vi "Test_MO.vi"() -> ()   [LabVIEW 2025]
panel:
  out "Valor 2":bool
  out "Valor":bool
  in  "Pin in":u8=4 min=4 max=40
  in  "Pin 3":u8=4 min=4 max=40
  in  "Pin 2":u8=4 min=4 max=40
  in  "Pin":u8=4 min=4 max=40
  in  "Estado 2":bool
  in  "stop":bool
  in  "VISA resource name":refnum<visa-resource-name>
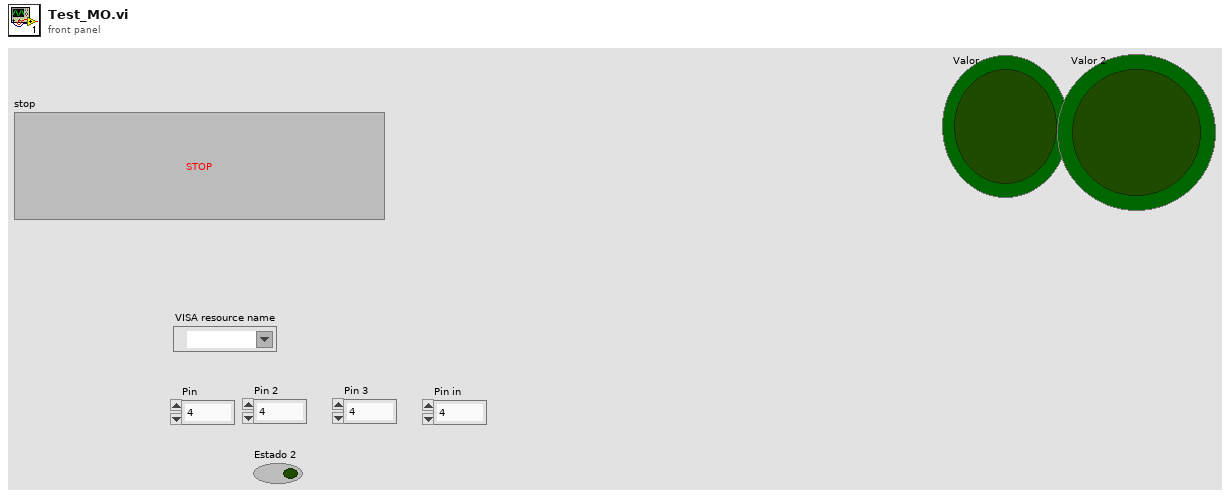
[diagram p1: front panel]
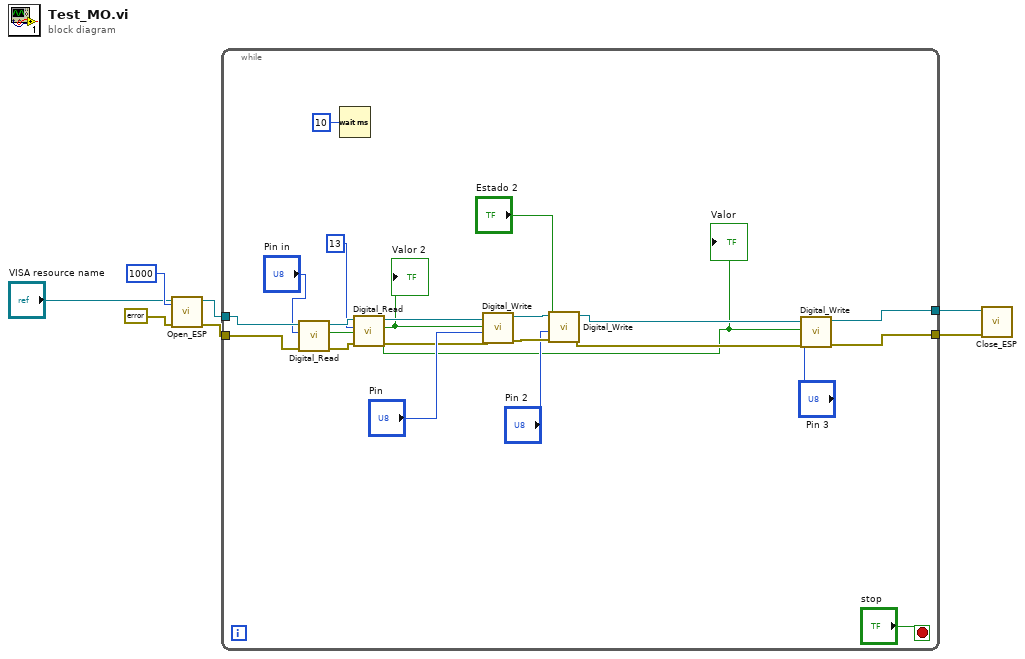
[diagram p0: block diagram]
diagram:
  n1 = call "Open_ESP.vi"("timeout (10sec)"=u32 1000, "error in (no error)"=errorcluster {"status"=FALSE, "code"=0, "source"=""}, "VISA resource name"="VISA resource name") -> ("error out"=w3:errorcluster, "VISA resource name out"=w4:refnum<visa-resource-name>)  [unwired: 7 in]
  n2 = while {
    tunnel: w4 -> [w17]
    tunnel: w3 -> [w16]
    tunnel: [w26] -> w2
    tunnel: [w25] -> w1
    stop <- "stop" stop-if-true
    n3 = call "Digital_Read.vi"("error in (no error)"=w16, "Pin"="Pin in", "VISA resource name"=w17) -> ("error out"=w10:errorcluster, "Valor"=w14:bool, "VISA resource name out"=w13:refnum<visa-resource-name>)  [unwired: 6 in]
    "Valor" <- w14
    n4 = Wait (ms)(milliseconds to wait=u32 10) -> ()  [unwired: 1 out]
    n5 = call "Digital_Read.vi"("error in (no error)"=w10, "Pin"=u8 13, "VISA resource name"=w13) -> ("error out"=w11:errorcluster, "Valor"=w8:bool, "VISA resource name out"=w12:refnum<visa-resource-name>)  [unwired: 6 in]
    "Valor 2" <- w8
    n6 = call "Digital_Write.vi"("error in (no error)"=w11, "Pin"="Pin", "Estado"=w8, "VISA resource name"=w12) -> ("error out"=w27:errorcluster, "VISA resource name out"=w24:refnum<visa-resource-name>)  [unwired: 6 in]
    n7 = call "Digital_Write.vi"("error in (no error)"=w27, "Pin"="Pin 2", "Estado"="Estado 2", "VISA resource name"=w24) -> ("error out"=w18:errorcluster, "VISA resource name out"=w19:refnum<visa-resource-name>)  [unwired: 6 in]
    n8 = call "Digital_Write.vi"("error in (no error)"=w18, "Pin"="Pin 3", "Estado"=w14, "VISA resource name"=w19) -> ("error out"=w26:errorcluster, "VISA resource name out"=w25:refnum<visa-resource-name>)  [unwired: 6 in]
  }
  n9 = call "Close_ESP.vi"("error in (no error)"=w2, "VISA resource name"=w1) -> ()  [unwired: 9 in, 1 out]
